vi "UHR-Fleezers Control (host) - 11.8.vi"() -> ()   [LabVIEW 2014] (continued)
        n2364 = call "reset FPGA DMA.vi"("error in"=w4799, "FPGA VI Reference In"=w4800) -> ("error out"=w4795:errorcluster, "FPGA VI Reference Out"=w4796:T19)
        n2365 = xnode "Read/Write Control"("FPGA VI Reference In"=w4796, "error in"=w4795, "AI to FIFO"=w4797, "APD to FIFO"=w4797) -> ("FPGA VI Reference Out"=w4794:T19, "error out"=w4793:errorcluster)
      }
    }
    n2366 = case shown="True" w3436 {
      frame False {
      }
      frame True {
        n2367 = local read "Flush rate (uL/m) P1"() -> (w3827:dbl)
        n2368 = local read "HP1 Flush Time (s)"() -> (w3833:dbl)
        n2369 = local read "DMA Update Period (s)"() -> (w3820:dbl)
        n2370 = Divide(x=w3827, y=60.0) -> (x/y=w3819:dbl)
        n2371 = feedback #4(0.0) -> (w3822:dbl)
        n2372 = Divide(x=w3833, y=w3820) -> (x/y=w3825:dbl)
        n2373 = feedback #5(0) -> (w3831:i32)
        n2374 = Increment(x=w3831) -> (x+1=w3824:i32)
        n2375 = Multiply(x=w3820, y=w3819) -> (x*y=w3818:dbl)
        n2376 = Greater?(x=w3824, y=w3825) -> (0:w3830:bool)
        n2377 = Compound Arithmetic op=MULTIPLY(w3820, w3824, w3819) -> (→"P1 Flush Volume (uL)":dbl)
        n2378 = Divide(x=w3824, y=w3825) -> (x/y=→"P1 Flushing Bar":dbl)
        n2379 = Add(x=w3818, y=w3822) -> (x+y=w3821:dbl)
        "Total Volume\nFlowed P1 (uL)" <- w3821
        n2380 = feedback-in #4(w3821) -> ()
        n2381 = case shown="True" w3830 {
          tunnel: w3824 -> [w3834 _]
          tunnel: [w3834 0] -> w3829
          frame False {
          }
          frame True {
            w3835 = FALSE ("Flushing P1")
            n2382 = local write "Inject Pump 1"(w3835) -> ()
            n2383 = local write "Flushing P1"(w3835) -> ()
            n2384 = property on="Clear Volume P1" class="Bool (strict)"("Val(Sgnl)"=TRUE ("Value (Signaling)")) -> ()  [unwired: 2 in, 2 out]
          }
        }
        n2385 = feedback-in #5(w3829) -> ()
      }
    }
    n2386 = Or(x="Start AOD Scan", y="Trap Raster Scan") -> (x .or. y?=w3671:bool)
    n2387 = case "Start AOM raster scan" shown="True" w3671 {
      tunnel: w3429 -> [w4642 w4652]
      tunnel: w3720 -> [w4641 w4651]
      tunnel: [w4642 w4645] -> w3719
      tunnel: [w4641 w4644] -> w3718
      frame False {
      }
      frame True {
        n2388 = case shown="True" "Restart DMA? (AOD)" {
          tunnel: [w4690 w4692] -> w4646
          tunnel: [w4689 w4691] -> w4647
          tunnel: w4652 -> [w4690 w4694]
          tunnel: w4651 -> [w4689 w4693]
          frame False {
          }
          frame True {
            n2389 = local write "Overflow (data lost)"(FALSE ("Overflow (data lost)")) -> ()
            n2390 = call "reset FPGA DMA.vi"("error in"=w4693, "FPGA VI Reference In"=w4694) -> ("error out"=w4691:errorcluster, "FPGA VI Reference Out"=w4692:T19)
          }
        }
        n2391 = local write "Trap Raster Scan"(FALSE ("Trap Raster Scan")) -> ()
        n2392 = case shown="False" "Move MCL Also?" {
          tunnel: w4647 -> [w4656 w4684]
          tunnel: w4646 -> [w4657 w4685]
          tunnel: [w4655 w4688] -> w4645
          tunnel: [w4654 w4687] -> w4644
          frame False {
            w4653 = TRUE ("AI to FIFO")
            n2393 = xnode "Read/Write Control"("FPGA VI Reference In"=w4657, "error in"=w4656, "AI to FIFO"=w4653, "APD to FIFO"=w4653, "Start scan"=w4653) -> ("FPGA VI Reference Out"=w4655:T19, "error out"=w4654:errorcluster)
          }
          frame True {
            w4681 = FALSE ("1D or 2D Scan?")
            w4686 = TRUE ("AI to FIFO")
            # "Count for MCL loop"
            # "N total cycles"
            # "N steps"
            # "V_int"
            n2394 = local read "Scan Range (nm)"() -> (w4663:dbl)
            n2395 = local read "Number of F/B Scans (AOD)"() -> (w4680:u16)
            n2396 = Sign(1:w4663) -> (0:w4662:dbl)
            n2397 = Compound Arithmetic op=MULTIPLY(w4663, "MCL Step Position Ratio", "MCL/AOM Scale Tweak") -> (w4667:dbl)
            n2398 = Negate(x=w4662) -> (-x=w4659:dbl)
            n2399 = Multiply(x=w4659, y="MCL Step Increment (V_int)") -> (x*y=w4661:dbl)
            n2400 = Divide(x=w4667, y="MCL X Cal (nm/V)") -> (x/y=w4673:dbl)
            n2401 = Multiply(x=32767.0 ("y"), y=w4673) -> (x*y=w4679:dbl)
            n2402 = local read "Total Counts (ticks)"() -> (w4664:u32)
            n2403 = local read "Cycles/step (AOD)"() -> (w4675:u64)
            n2404 = local read "Scan steps (AOD)"() -> (w4676:u64)
            n2405 = Divide(x=w4679, y=10.0) -> (x/y=w4672:dbl)
            n2406 = Divide(x=w4672, y="MCL Step Increment (V_int)") -> (x/y=w4670:dbl)
            n2407 = Absolute Value(x=w4670) -> (abs(x)=w4658:dbl)
            n2408 = Compound Arithmetic op=MULTIPLY(w4676, w4675, w4664) -> (w4671:u64)
            n2409 = local write "wait to reset values"(w4686) -> ()
            n2410 = local write "MCL Scanning"(w4686) -> ()
            n2411 = Divide(x=w4671, y=w4658) -> (x/y=w4668:dbl)
            "MCL Count" <- w4668
            n2412 = xnode "Read/Write Control"("FPGA VI Reference In"=w4685, "error in"=w4684, "Scan steps (MCL)"=w4658, "Number of scans (MCL)"=w4680, "Cycles per step (MCL)"=u64 1, "Scan freq.  increment (MCL)"=w4661, "1D or 2D Scan?"=w4681, "MCL Scan Axis"=w4681, "Cont. Scan (MCL)"=w4681, "MCL count"=w4668) -> ("FPGA VI Reference Out"=w4683:T19, "error out"=w4682:errorcluster)
            n2413 = xnode "Read/Write Control"("FPGA VI Reference In"=w4683, "error in"=w4682, "AI to FIFO"=w4686, "APD to FIFO"=w4686, "Start scan"=w4686, "Start scan (MCL)"=w4686) -> ("FPGA VI Reference Out"=w4688:T19, "error out"=w4687:errorcluster)
          }
        }
        "Raster Scanning..." <- TRUE ("Scanning...")
      }
    }
    n2414 = local read "Flushing P3"() -> (w3437:bool)
    n2415 = case "Keep track of when Harvard Pump 3 is done flushing" shown="True" w3437 {
      frame False {
      }
      frame True {
        n2416 = local read "Flush rate (uL/m) P3"() -> (w3846:dbl)
        n2417 = local read "DMA Update Period (s)"() -> (w3840:dbl)
        n2418 = local read "HP3 Flush Time (s)"() -> (w3854:dbl)
        n2419 = Divide(x=w3846, y=60.0) -> (x/y=w3841:dbl)
        n2420 = feedback #6(0) -> (w3852:i32)
        n2421 = Increment(x=w3852) -> (x+1=w3847:i32)
        n2422 = Divide(x=w3854, y=w3840) -> (x/y=w3848:dbl)
        n2423 = Multiply(x=w3840, y=w3841) -> (x*y=w3839:dbl)
        n2424 = Greater?(x=w3847, y=w3848) -> (0:w3851:bool)
        n2425 = feedback #7(0.0) -> (w3842:dbl)
        n2426 = Compound Arithmetic op=MULTIPLY(w3840, w3847, w3841) -> (→"P3 Flush Volume (uL)":dbl)
        n2427 = case shown="True" w3851 {
          tunnel: w3847 -> [w3855 _]
          tunnel: [w3855 0] -> w3850
          frame False {
          }
          frame True {
            w3856 = FALSE ("Flushing P3")
            n2428 = local write "Inject Pump 3"(w3856) -> ()
            n2429 = local write "Flushing P3"(w3856) -> ()
            n2430 = property on="Clear Volume P3" class="Bool (strict)"("Val(Sgnl)"=TRUE ("Value (Signaling)")) -> ()  [unwired: 2 in, 2 out]
          }
        }
        n2431 = feedback-in #6(w3850) -> ()
        n2432 = Divide(x=w3847, y=w3848) -> (x/y=→"P3 Flushing Bar":dbl)
        n2433 = Add(x=w3839, y=w3842) -> (x+y=w3843:dbl)
        "Total Volume\nFlowed P3 (uL)" <- w3843
        n2434 = feedback-in #7(w3843) -> ()
      }
    }
    n2435 = And(x="Save scans", y=w3671) -> (x .and. y?=w3717:bool)
    n2436 = local read "Flushing samp"() -> (w3430:bool)
    n2437 = case shown="True" w3430 {
      frame False {
      }
      frame True {
        n2438 = local read "DMA Update Period (s)"() -> (w3799:dbl)
        n2439 = local read "Flush rate (mL/m)"() -> (w3811:dbl)
        n2440 = local read "Samp Flush Time (s)"() -> (w3812:dbl)
        n2441 = Divide(x=w3811, y=60.0) -> (x/y=w3798:dbl)
        n2442 = feedback #8(0) -> (w3804:i32)
        n2443 = Increment(x=w3804) -> (x+1=w3803:i32)
        n2444 = Divide(x=w3812, y=w3799) -> (x/y=w3808:dbl)
        n2445 = Multiply(x=w3799, y=w3798) -> (x*y=w3797:dbl)
        n2446 = Greater?(x=w3803, y=w3808) -> (0:w3807:bool)
        n2447 = feedback #9(0.0) -> (w3800:dbl)
        n2448 = Compound Arithmetic op=MULTIPLY(w3799, w3803, w3798) -> (→"Samp Volume (uL)":dbl)
        n2449 = Divide(x=w3803, y=w3808) -> (x/y=→"Samp flush bar":dbl)
        n2450 = case shown="True" w3807 {
          tunnel: [w3813 0] -> w3806
          tunnel: w3803 -> [w3813 _]
          frame False {
          }
          frame True {
            w3816 = FALSE ("Flushing samp")
            n2451 = local write "Sample Channel\nFlow"(w3816) -> ()
            n2452 = local write "Flushing samp"(w3816) -> ()
            n2453 = property on="Clear Volume" class="Bool (strict)"("Val(Sgnl)"=TRUE) -> ()  [unwired: 2 in, 2 out]
          }
        }
        n2454 = feedback-in #8(w3806) -> ()
        n2455 = Add(x=w3797, y=w3800) -> (x+y=w3801:dbl)
        "Total Volume\nFlowed Samp (uL)" <- w3801
        n2456 = feedback-in #9(w3801) -> ()
      }
    }
    n2457 = Compound Arithmetic op=OR("Start MCL Scan", "Confocal\nImage", "Confocal\nLinescan") -> (w3669:bool)
    n2458 = And(x="Save Data (MCL)", y=w3669) -> (x .and. y?=w3716:bool)
    n2459 = case "Start MCL raster scan" shown="True" w3669 {
      tunnel: w3719 -> [w4259 w4275]
      tunnel: w3718 -> [w4258 w4274]
      tunnel: [w4259 w4270] -> w3428
      tunnel: [w4258 w4269] -> w3426
      tunnel: [FALSE w4268] -> w3702
      tunnel: "Start MCL Scan" -> [_ w4263]
      tunnel: "Confocal\nImage" -> [_ w4262]
      tunnel: "Confocal\nLinescan" -> [_ _]
      frame False {
      }
      frame True {
        w4268 = TRUE
        n2460 = case shown="True" "Restart DMA? (MCL)" {
          tunnel: [w4320 w4322] -> w4273
          tunnel: [w4319 w4321] -> w4272
          tunnel: w4275 -> [w4320 w4325]
          tunnel: w4274 -> [w4319 w4324]
          frame False {
          }
          frame True {
            n2461 = call "reset FPGA DMA.vi"("error in"=w4324, "FPGA VI Reference In"=w4325) -> ("error out"=w4321:errorcluster, "FPGA VI Reference Out"=w4322:T19)
            n2462 = local write "Overflow (data lost)"(FALSE ("Overflow (data lost)")) -> ()
          }
        }
        n2463 = case shown="False" w4263 {
          selector: w4263 -> [_ w4279]
          tunnel: w4262 -> [w4278 _]
          tunnel: [w4278 w4279] -> w4261
          frame False {
            n2464 = property on="2D or 1D Scan" class="Bool (strict)"("Val(Sgnl)"=w4278) -> ()  [unwired: 2 in, 2 out]
            n2465 = property on="Confocal\nImage" class="Bool (strict)"("Value"=FALSE ("Start Confocal Map")) -> ()  [unwired: 2 in, 2 out]
          }
          frame True {
          }
        }
        n2466 = local write "MCL Scanning"(w4268) -> ()
        n2467 = local read "AO1"() -> (w4265:dbl)
        n2468 = local read "AO2"() -> (w4264:dbl)
        n2469 = case shown="True" "Center Scan" {
          tunnel: w4273 -> [w4286 w4318]
          tunnel: w4272 -> [w4285 w4317]
          tunnel: [w4284 w4316] -> w4270
          tunnel: [w4283 w4315] -> w4269
          tunnel: [w4281 w4302] -> w4267
          tunnel: [w4280 w4301] -> w4266
          tunnel: w4265 -> [w4281 w4307]
          tunnel: w4264 -> [w4280 w4310]
          tunnel: w4261 -> [_ _]
          frame False {
            w4282 = TRUE ("AI to FIFO")
            n2470 = xnode "Read/Write Control"("FPGA VI Reference In"=w4286, "error in"=w4285, "AI to FIFO"=w4282, "APD to FIFO"=w4282, "Start scan (MCL)"=w4282) -> ("FPGA VI Reference Out"=w4284:T19, "error out"=w4283:errorcluster)
          }
          frame True {
            w4314 = TRUE ("AI to FIFO")
            n2471 = local read "Scan steps (MCL)"() -> (w4293:u64)
            n2472 = local read "Scan lines (y)"() -> (w4289:u64)
            n2473 = local read "Fast Scan Dir"() -> (w4300:bool)
            n2474 = local read "Actual MCL Inc (V)"() -> (w4290:dbl)
            n2475 = Decrement(x=w4289) -> (x-1=w4288:u64)
            n2476 = Decrement(x=w4293) -> (x-1=w4292:u64)
            n2477 = Multiply(x=w4290, y=w4288) -> (x*y=w4287:dbl)
            n2478 = Divide(x=w4287, y=2.0) -> (x/y=w4297:dbl)
            n2479 = Multiply(x=w4290, y=w4292) -> (x*y=w4291:dbl)
            n2480 = Divide(x=w4291, y=2.0) -> (x/y=w4296:dbl)
            n2481 = Select(t=w4296, s=w4300, f=w4297) -> (s? t:f=w4295:dbl)
            n2482 = Select(t=w4297, s=w4300, f=w4296) -> (s? t:f=w4299:dbl)
            n2483 = Subtract(x=w4307, y=w4299) -> (x-y=w4298:dbl)
            n2484 = Subtract(x=w4310, y=w4295) -> (x-y=w4294:dbl)
            n2485 = local read "2D or 1D Scan"() -> (w4312:bool)
            n2486 = Not(x=w4300) -> (.not. x?=w4306:bool)
            n2487 = Not(x=w4312) -> (.not. x?=w4308:bool)
            n2488 = And(x=w4300, y=w4308) -> (x .and. y?=w4309:bool)
            n2489 = And(x=w4308, y=w4306) -> (x .and. y?=w4311:bool)
            n2490 = Select(t=w4310, s=w4311, f=w4294) -> (s? t:f=w4301:dbl)
            n2491 = Select(t=w4307, s=w4309, f=w4298) -> (s? t:f=w4302:dbl)
            n2492 = call "Volt to I16.vi"("Voltage In"=w4302) -> ("I16 Voltage Out"=w4305:i16)
            n2493 = call "Volt to I16.vi"("Voltage In"=w4301) -> ("I16 Voltage Out"=w4304:i16)
            n2494 = xnode "Read/Write Control"("FPGA VI Reference In"=w4318, "error in"=w4317, "AI to FIFO"=w4314, "APD to FIFO"=w4314, "Start scan (MCL)"=w4314, "AO1"=w4305, "AO2"=w4304) -> ("FPGA VI Reference Out"=w4316:T19, "error out"=w4315:errorcluster)
          }
        }
        "Initial Y" <- w4267
        "Initial X" <- w4266
        n2495 = local write "Tab Control 6"(T3."Imaging" ("Tab Control 6")) -> ()
        "wait to reset values" <- w4268
      }
    }
    n2496 = case shown="True" "Wiggle" {
      selector: "Wiggle" -> [w3770 _]
      tunnel: w3428 -> [w3772 w3785]
      tunnel: [w3769 w3788] -> w3427
      tunnel: w3426 -> [w3771 w3783]
      tunnel: [w3768 w3787] -> w3425
      frame False {
        n2497 = xnode "Read/Write Control"("FPGA VI Reference In"=w3772, "error in"=w3771, "Wiggle trap 1"=w3770) -> ("FPGA VI Reference Out"=w3769:T19, "error out"=w3768:errorcluster)
      }
      frame True {
        w3777 = FALSE ("Abort wiggle")
        w3781 = TRUE
        n2498 = local read "Restart DMA? (AOD)"() -> (w3786:bool)
        n2499 = case shown="True" w3786 {
          tunnel: w3785 -> [w3790 w3795]
          tunnel: [w3790 w3794] -> w3784
          tunnel: w3783 -> [w3789 w3793]
          tunnel: [w3789 w3792] -> w3782
          frame False {
          }
          frame True {
            n2500 = local write "Overflow (data lost)"(FALSE) -> ()
            n2501 = call "reset FPGA DMA.vi"("error in"=w3793, "FPGA VI Reference In"=w3795) -> ("error out"=w3792:errorcluster, "FPGA VI Reference Out"=w3794:T19)
          }
        }
        n2502 = local write "Wiggle"(FALSE) -> ()
        n2503 = xnode "Read/Write Control"("FPGA VI Reference In"=w3784, "error in"=w3782, "AI to FIFO"=w3781, "APD to FIFO"=w3781, "Wiggle trap 1"="Wiggle T1", "Wiggle freq 1 (Hz)"="Wiggle freq 1 (Hz)", "Wiggle amp 1"="Wiggle amp 1 (units?)", "Abort wiggle 1"=w3777, "Wiggle trap 2"="Wiggle T2", "Abort wiggle 2"=w3777, "Wiggle freq 2 (Hz)"="Wig Freq 2 (Hz)", "Wiggle amp 2"="Wig amp 2") -> ("FPGA VI Reference Out"=w3788:T19, "error out"=w3787:errorcluster)
      }
    }
    n2504 = local read "Trap Pos Elements/DMA read"() -> (w3559:u32)
    n2505 = local read "Trap AI Elements/DMA read"() -> (w3632:u32)
    n2506 = local read "APD Elements/DMA read"() -> (w3598:u32)
    n2507 = xnode "Get APD Data"("FPGA VI Reference In"=w3427, "error in"=w3425, "Number of Elements"=w3598, "Timeout (ms)"=-1) -> ("Data"=w3597:u32[], "Elements Remaining"=→"APD FIFO Elements Remaining":u32)  [unwired: 2 out]
    n2508 = xnode "Invoke Method"("FPGA VI Reference In"=w3427, "error in"=w3425, "Number of Elements"=w3559, "Timeout (ms)"=-1) -> ("Data"=w3523:u16[], "Elements Remaining"=→"Trap Pos FIFO El Remaining":u32)  [unwired: 2 out]
    n2509 = xnode "Get Trap Data"("FPGA VI Reference In"=w3427, "error in"=w3425, "Number of Elements"=w3632, "Timeout (ms)"=-1 ("Timeout")) -> ("FPGA VI Reference Out"=w3458:T19, "error out"=w3457:errorcluster, "Data"=w3524:i16[], "Elements Remaining"=w3762:u32)
    "FIFO El. Rem." <- w3762
    n2510 = local read "Trap AI FIFO Depth"() -> (w3764:u32)
    n2511 = Subtract(x=w3764, y=w3632) -> (x-y=w3763:u32)
    n2512 = Decimate 1D Array(w3523) -> (w3520:u16[], w3522:u16[], w3521:u16[])
    n2513 = Divide(x=w3762, y=w3763) -> (x/y=w3761:dbl)
    "Buffer Status" <- w3761
    n2514 = To Unsigned Long Integer(number=w3520) -> (unsigned 32bit integer=w3519:u32[])
    n2515 = Join Numbers(hi=w3522, lo=w3521) -> ((hi.lo)=w3518:u32[])
    n2516 = Equal?(x=w3761, y=1.0) -> (x = y?=w3759:bool)
    n2517 = Join Numbers(hi=w3519, lo=w3518) -> ((hi.lo)=w3512:u64[])
    n2518 = call "IR AOM word to freq - vec.vi"("Frequency Word In (double vec)"=w3512) -> ("Frequency Out"=w3558:dbl[])
    n2519 = case "Alert buffer overflow" shown="True" w3759 {
      frame False {
      }
      frame True {
        n2520 = call <vilib>:"Beep.vi"() -> ()  [unwired: 3 in, 9 out]
        "Overflow (data lost)" <- TRUE ("Overflow (data lost)")
      }
    }
    n2521 = Decimate 1D Array(w3558) -> (w3557:dbl[], w3556:dbl[])
    n2522 = Build Array(w3557, w3556) -> (w3555:dbl[][])
    n2523 = local read "Trap Sets"() -> (w3631:u32)
    n2524 = case "Deinterlace trap data, average down PSD" shown="2" w3631 {
      tunnel: w3524 -> [w4355 w4420]
      tunnel: [w4352 w4417] -> w3624
      tunnel: [w4355 w4419] -> w3515
      tunnel: "Detector Type" -> [w4354 w4415]
      tunnel: [w4353 w4418] -> w3623
      tunnel: [w4351 w4416] -> w3736
      frame 1, Default {
        n2525 = Divide(x=w4355, y=3276.7) -> (x/y=w4356:dbl[])
        n2526 = Decimate 1D Array(w4356) -> (w4365:dbl[], w4364:dbl[], w4363:dbl[], w4362:dbl[], w4361:dbl[], w4360:dbl[], w4359:dbl[], w4358:dbl[])
        n2527 = case shown="\"IR-QPD + PSD + FB-QPD position\"" w4354 {
          tunnel: w4365 -> [w4389 w4414]
          tunnel: w4364 -> [w4388 w4413]
          tunnel: w4363 -> [w4373 w4391]
          tunnel: w4362 -> [w4374 w4401]
          tunnel: w4361 -> [w4387 w4412]
          tunnel: w4360 -> [w4386 w4411]
          tunnel: w4359 -> [w4370 w4392]
          tunnel: w4358 -> [w4369 w4390]
          tunnel: [w4368 w4398] -> w4353
          tunnel: [w4367 w4397] -> w4352
          tunnel: [w4366 w4396] -> w4351
          frame "IR-QPD + PSD + FB-QPD", Default {
            w4366 = 0  # Channel pattern
            n2528 = Divide(x=w4389, y=w4374) -> (x/y=w4376:dbl[])
            n2529 = Divide(x=w4388, y=w4374) -> (x/y=w4375:dbl[])
            n2530 = Divide(x=w4387, y=w4370) -> (x/y=w4372:dbl[])
            n2531 = Divide(x=w4386, y=w4369) -> (x/y=w4371:dbl[])
            n2532 = Build Array(w4376, w4375, w4374, w4373, w4372, w4371, w4370, w4369) -> (w4367:dbl[][])
            n2533 = Bundle("T1 Y", "T1 X", "T1 Sum", "FB Sum", "PSD Y", "PSD X", "PSD Y Sum", "PSD X Sum") -> (w4385:T41)  [unwired: 1 out]
            n2534 = Cluster To Array(cluster=w4385) -> (array=w4368:string[])
          }
          frame "IR-QPD + PSD + FB-QPD position" {
            w4396 = 3  # Channel pattern
            n2535 = Negate(x=w4392) -> (-x=w4393:dbl[])
            n2536 = Divide(x=w4414, y=w4401) -> (x/y=w4403:dbl[])
            n2537 = Divide(x=w4413, y=w4401) -> (x/y=w4402:dbl[])
            n2538 = Divide(x=w4412, y=w4392) -> (x/y=w4400:dbl[])
            n2539 = Divide(x=w4411, y=w4393) -> (x/y=w4399:dbl[])
            n2540 = Build Array(w4403, w4402, w4401, w4390, w4391, w4400, w4399, w4392) -> (w4397:dbl[][])
            n2541 = Bundle("T1 Y", "T1 X", "T1 Sum", "FB X", "FB Sum", "PSD Y", "PSD X", "PSD Y Sum") -> (w4410:T41)  [unwired: 1 out]
            n2542 = Cluster To Array(cluster=w4410) -> (array=w4398:string[])
          }
        }
      }
      frame 2 {
        n2543 = case shown="\"IR-QPD + PSD + FB-QPD\", Default" w4415 {
          tunnel: w4420 -> [w4482 w4549 w4620]
          tunnel: [w4421 w4540 w4551] -> w4419
          tunnel: [w4448 w4531 w4598] -> w4418
          tunnel: [w4447 w4494 w4565] -> w4417
          tunnel: [w4441 w4529 w4596] -> w4416
          frame "IR-QPD + PSD + FB-QPD", Default {
            w4441 = 1  # Channel pattern
            # "time average x2 the 4th signal and the 4 psd signals (detection laser)"
            # "deinterlace 3 signals from qpd"
            n2544 = Decimate 1D Array(w4482) -> (w4481:i16[], w4480:i16[], w4446:i16[], w4479:i16[], w4469:i16[], w4467:i16[], w4466:i16[], w4464:i16[])
            n2545 = Decimate 1D Array(w4446) -> (w4445:i16[], w4444:i16[])
            n2546 = Decimate 1D Array(w4481) -> (w4478:i16[], w4450:i16[])
            n2547 = Decimate 1D Array(w4480) -> (w4477:i16[], w4475:i16[])
            n2548 = Decimate 1D Array(w4479) -> (w4476:i16[], w4474:i16[])
            n2549 = call "downsample 1D array - double.vi"("Ave N"=2.0, "Array In"=w4469) -> ("Array Out"=w4468:dbl[])  [unwired: 1 out]
            n2550 = call "downsample 1D array - double.vi"("Ave N"=2.0, "Array In"=w4467) -> ("Array Out"=w4449:dbl[])  [unwired: 1 out]
            n2551 = call "downsample 1D array - double.vi"("Ave N"=2.0, "Array In"=w4466) -> ("Array Out"=w4465:dbl[])  [unwired: 1 out]
            n2552 = call "downsample 1D array - double.vi"("Ave N"=2.0, "Array In"=w4464) -> ("Array Out"=w4463:dbl[])  [unwired: 1 out]
            n2553 = Interleave 1D Arrays(w4478, w4477, w4476, w4450, w4475, w4474, w4445, w4444, w4468, w4449, w4465, w4463) -> (w4462:dbl[])
            n2554 = Divide(x=w4462, y=3276.7) -> (x/y=w4461:dbl[])
            n2555 = Decimate 1D Array(w4461) -> (w4460:dbl[], w4459:dbl[], w4458:dbl[], w4457:dbl[], w4456:dbl[], w4455:dbl[], w4443:dbl[], w4442:dbl[], w4454:dbl[], w4453:dbl[], w4452:dbl[], w4451:dbl[])
            n2556 = Divide(x=w4460, y=w4458) -> (x/y=w4428:dbl[])
            n2557 = Divide(x=w4459, y=w4458) -> (x/y=w4427:dbl[])
            n2558 = Divide(x=w4457, y=w4455) -> (x/y=w4426:dbl[])
            n2559 = Divide(x=w4456, y=w4455) -> (x/y=w4425:dbl[])
            n2560 = Divide(x=w4454, y=w4452) -> (x/y=w4424:dbl[])
            n2561 = Divide(x=w4453, y=w4451) -> (x/y=w4423:dbl[])
            n2562 = Build Array(w4428, w4427, w4458, w4426, w4425, w4455, w4443, w4442, w4424, w4423, w4452, w4451) -> (w4447:dbl[][])
            n2563 = Bundle("T1 Y", "T1 X", "T1 Sum", "T2 Y", "T2 X", "T2 Sum", "T1 FB Sum", "T2 FB Sum", "PSD Y", "PSD X", "PSD Y Sum", "PSD X Sum") -> (w4429:T42)  [unwired: 1 out]
            n2564 = To Word Integer(number=w4462) -> (16bit integer=w4421:i16[])
            n2565 = Cluster To Array(cluster=w4429) -> (array=w4448:string[])
          }
          frame "IR-QPD + PSD + FB-QPD X position" {
            w4529 = 2  # Channel pattern
            # "time average x2 the 3 psd signals (detection laser)"
            # "deinterlace 3 signals from qpds"
            n2566 = Decimate 1D Array(w4549) -> (w4548:i16[], w4547:i16[], w4530:i16[], w4546:i16[], w4492:i16[], w4489:i16[], w4486:i16[], w4517:i16[])
            n2567 = Decimate 1D Array(w4530) -> (w4515:i16[], w4513:i16[])
            n2568 = Decimate 1D Array(w4548) -> (w4545:i16[], w4532:i16[])
            n2569 = Decimate 1D Array(w4547) -> (w4544:i16[], w4542:i16[])
            n2570 = Decimate 1D Array(w4546) -> (w4543:i16[], w4541:i16[])
            n2571 = Decimate 1D Array(w4517) -> (w4516:i16[], w4514:i16[])
            n2572 = call "downsample 1D array - I16.vi"("Ave N"=2.0, "Array In"=w4492) -> ("Array Out"=w4490:i16[])  [unwired: 1 in]
            n2573 = call "downsample 1D array - I16.vi"("Ave N"=2.0, "Array In"=w4486) -> ("Array Out"=w4484:i16[])  [unwired: 1 in]
            n2574 = call "downsample 1D array - I16.vi"("Ave N"=2.0, "Array In"=w4489) -> ("Array Out"=w4487:i16[])  [unwired: 1 in]
            n2575 = Interleave 1D Arrays(w4545, w4544, w4543, w4532, w4542, w4541, w4516, w4515, w4514, w4513, w4490, w4487, w4484) -> (w4540:i16[])
            n2576 = Divide(x=w4540, y=3276.7) -> (x/y=w4539:dbl[])
            n2577 = Decimate 1D Array(w4539) -> (w4538:dbl[], w4537:dbl[], w4536:dbl[], w4535:dbl[], w4534:dbl[], w4533:dbl[], w4505:dbl[], w4503:dbl[], w4502:dbl[], w4500:dbl[], w4499:dbl[], w4498:dbl[], w4495:dbl[])
            n2578 = Negate(x=w4495) -> (-x=w4493:dbl[])
            n2579 = Divide(x=w4499, y=w4495) -> (x/y=w4497:dbl[])
            n2580 = Divide(x=w4498, y=w4493) -> (x/y=w4496:dbl[])
            n2581 = Divide(x=w4538, y=w4536) -> (x/y=w4521:dbl[])
            n2582 = Divide(x=w4537, y=w4536) -> (x/y=w4520:dbl[])
            n2583 = Divide(x=w4535, y=w4533) -> (x/y=w4519:dbl[])
            n2584 = Divide(x=w4534, y=w4533) -> (x/y=w4518:dbl[])
            n2585 = Divide(x=w4505, y=w4503) -> (x/y=w4504:dbl[])
            n2586 = Divide(x=w4502, y=w4500) -> (x/y=w4501:dbl[])
            n2587 = Build Array(w4521, w4520, w4536, w4519, w4518, w4533, w4504, w4503, w4501, w4500, w4497, w4496, w4495) -> (w4494:dbl[][])
            n2588 = Bundle("T1 Y", "T1 X", "T1 Sum", "T2 Y", "T2 X", "T2 Sum", "T1 FB X", "T1 FB Sum", "T2 FB X", "T2 FB Sum", "PSD Y", "PSD X", "PSD Y Sum") -> (w4522:T43)  [unwired: 1 out]
            n2589 = Cluster To Array(cluster=w4522) -> (array=w4531:string[])
          }
          frame "IR-QPD + PSD + FB-QPD XY positions" {
            w4596 = 4  # Channel pattern
            # "time average x2 the 3 psd signals (detection laser)"
            # "deinterlace 3 signals from qpds"
            n2590 = Decimate 1D Array(w4620) -> (w4619:i16[], w4618:i16[], w4597:i16[], w4617:i16[], w4563:i16[], w4609:i16[], w4608:i16[], w4585:i16[])
            n2591 = Decimate 1D Array "Feedback Sum"(w4597) -> (w4581:i16[], w4579:i16[])
            n2592 = Decimate 1D Array "QPD Y"(w4619) -> (w4616:i16[], w4599:i16[])
            n2593 = Decimate 1D Array "QPD X"(w4618) -> (w4615:i16[], w4613:i16[])
            n2594 = Decimate 1D Array "Feedback Y"(w4563) -> (w4562:i16[], w4561:i16[])
            n2595 = Decimate 1D Array "QPD Sum"(w4617) -> (w4614:i16[], w4612:i16[])
            n2596 = Decimate 1D Array "Feedback X"(w4585) -> (w4582:i16[], w4580:i16[])
            n2597 = call "downsample 1D array - double.vi"("Ave N"=2.0, "Array In"=w4609) -> ("Array Out"=w4584:dbl[])  [unwired: 1 out]
            n2598 = call "downsample 1D array - double.vi"("Ave N"=2.0, "Array In"=w4608) -> ("Array Out"=w4583:dbl[])  [unwired: 1 out]
            n2599 = Interleave 1D Arrays(w4616, w4615, w4614, w4599, w4613, w4612, w4562, w4582, w4581, w4561, w4580, w4579, w4584, w4583) -> (w4607:dbl[])
            n2600 = Divide(x=w4607, y=3276.7) -> (x/y=w4606:dbl[])
            n2601 = Decimate 1D Array(w4606) -> (w4605:dbl[], w4604:dbl[], w4603:dbl[], w4602:dbl[], w4601:dbl[], w4600:dbl[], w4558:dbl[], w4572:dbl[], w4556:dbl[], w4557:dbl[], w4570:dbl[], w4554:dbl[], w4568:dbl[], w4566:dbl[])
            n2602 = Negate(x=w4566) -> (-x=w4564:dbl[])
            n2603 = Divide(x=w4568, y=w4564) -> (x/y=w4567:dbl[])
            n2604 = Divide(x=w4557, y=w4554) -> (x/y=w4553:dbl[])
            n2605 = Divide(x=w4558, y=w4556) -> (x/y=w4555:dbl[])
            n2606 = Divide(x=w4605, y=w4603) -> (x/y=w4589:dbl[])
            n2607 = Divide(x=w4604, y=w4603) -> (x/y=w4588:dbl[])
            n2608 = Divide(x=w4602, y=w4600) -> (x/y=w4587:dbl[])
            n2609 = Divide(x=w4601, y=w4600) -> (x/y=w4586:dbl[])
            n2610 = Divide(x=w4572, y=w4556) -> (x/y=w4571:dbl[])
            n2611 = Divide(x=w4570, y=w4554) -> (x/y=w4569:dbl[])
            n2612 = Build Array(w4589, w4588, w4603, w4587, w4586, w4600, w4555, w4571, w4556, w4553, w4569, w4554, w4567, w4566) -> (w4565:dbl[][])
            n2613 = Bundle("T1 Y", "T1 X", "T1 Sum", "T2 Y", "T2 X", "T2 Sum", "T1 FB Y", "T1 FB X", "T1 FB Sum", "T2 FB Y", "T2 FB X", "T2 FB Sum", "PSD X", "PSD Y Sum") -> (w4552:T44)  [unwired: 1 out]
            n2614 = To Word Integer(number=w4607) -> (16bit integer=w4551:i16[])
            n2615 = Cluster To Array(cluster=w4552) -> (array=w4598:string[])
          }
        }
      }
    }
    "AI labels" <- w3623
    n2616 = Decimate 1D Array(w3597) -> (w3621:u32[], w3565:u32[])
    n2617 = local read "DMA Update Period (s)"() -> (w3633:dbl)
    n2618 = Build Array(w3621, w3565) -> (w3699:u32[][])
    n2619 = local read "Data Period (s)"() -> (w3474:dbl)
    n2620 = local read "BD 1 Frequency 2 (MHz)"() -> (w3507:dbl)
    n2621 = local read "BD 1 Frequency 1 (MHz)"() -> (w3508:dbl)
    n2622 = Decimate 1D Array(w3515) -> (w3538:i16[], w3537:i16[], w3535:i16[], w3534:i16[])  [unwired: 9 out]
    n2623 = To Double Precision Float(number=w3699) -> (double precision float=w3700:dbl[][])
    n2624 = local read "APD Integration Time (s)"() -> (w3578:dbl)
    n2625 = Multiply(x=w3474, y="Trap Pos. Disp. Downsample") -> (x*y=w3472:dbl)
    n2626 = Divide(x=w3538, y=w3537) -> (x/y=w3539:dbl[])
    n2627 = Divide(x=w3535, y=w3534) -> (x/y=w3536:dbl[])
    n2628 = feedback #10(0.0) -> (w3552:dbl)
    n2629 = Add(x=w3633, y=w3552) -> (x+y=w3738:dbl)
    n2630 = feedback-in #10(w3738) -> ()
    n2631 = local read "AOM X Cal (nm/MHz)"() -> (w3505:dbl)
    n2632 = To Time Stamp(1:w3552) -> (0:w3551:timestamp)
    n2633 = Split 1D Array(array=w3539, index="N El. to Ave.") -> (second subarray=w3542:dbl[])  [unwired: 1 out]
    n2634 = Split 1D Array(array=w3536, index="N El. to Ave.") -> (second subarray=w3541:dbl[])  [unwired: 1 out]
    n2635 = Multiply(x=w3474, y="Trap Disp. Downsample") -> (x*y=w3553:dbl)
    "Display Period (s)" <- w3553
    n2636 = for "Trap AI" {
      tunnel: [w4350] -> w3732 mode=indexing
      tunnel: w3551 -> [w4340]
      tunnel: "Trap Disp. Downsample" -> [w4348]
      tunnel: w3624 -> [w4346] mode=indexing
      tunnel: w3474 -> [w4345]
      tunnel: w3623 -> [w4344] mode=indexing
      tunnel: w3550 -> [w4343]
      tunnel: [w4342] -> w3589 mode=indexing
      tunnel: w3553 -> [w4341]
      workers-P: _ -> [_]
      n2637 = Bundle By Name("Y"=w4346, "dt"=w4345) -> (w4347:waveform(dbl))  [unwired: 1 out]
      n2638 = Set Waveform Attribute(5:w4344, 6:w4343, 7:w4347) -> (3:w4342:waveform(dbl))  [unwired: 1 in, 2 out]
      n2639 = call "downsample 1D array - double.vi"("Ave N"=w4348, "Array In"=w4346) -> ("Array Out"=w4349:dbl[])  [unwired: 1 out]
      n2640 = Bundle By Name(cluster=w4342, "t0"=w4340, "Y"=w4349, "dt"=w4341) -> (w4350:waveform(dbl))
    }
    n2641 = Bundle("BD 1 Frequency 1 (MHz)"=w3508, "BD 1 Frequency 2 (MHz)"=w3507) -> (w3509:T45)  [unwired: 1 out]
    n2642 = call-poly <vilib>:"Mean.vi"("X"=w3541) -> ("mean"=w3529:dbl)  [unwired: 1 out]
    n2643 = call-poly <vilib>:"Mean.vi"("X"=w3542) -> ("mean"=w3530:dbl)  [unwired: 1 out]
    n2644 = Reciprocal(x=w3553) -> (1/x=→"Trap Disp. Freq. (Hz)":dbl)
    n2645 = Cluster To Array(cluster=w3509) -> (array=w3506:dbl[])
    n2646 = local read "Trap X AI1 (DMA)"() -> (w3540:T13)
    n2647 = local read "Data points/scans (MCL)"() -> (w3711:dbl)
    n2648 = To Fixed-Point(number=w3529) -> (fixed-point=w3527:fxp<+/-,16,1>)  [unwired: 1 in]
    n2649 = To Fixed-Point(number=w3530) -> (fixed-point=w3528:fxp<+/-,16,1>)  [unwired: 1 in]
    n2650 = Bundle("Trap 1 Pos.", "Trap 2 Pos.") -> (w3549:cluster{string, string})  [unwired: 1 out]
    n2651 = Bundle By Name(cluster=w3540, "Set 1"=w3528, "Set 2"=w3527) -> (→"Trap X AI1 (DMA)":T13)
    n2652 = Cluster To Array(cluster=w3549) -> (array=w3546:string[])
    n2653 = Bundle("APD 1", "APD 2") -> (w3731:cluster{string, string})  [unwired: 1 out]
    n2654 = Select(t=-1.0, s="Negate Y Axis", f=1.0) -> (s? t:f=w3491:dbl)
    n2655 = for "Trap Position" {
      tunnel: w3555 -> [w3984] mode=indexing
      tunnel: "Trap Pos. Disp. Downsample" -> [w3983]
      tunnel: w3472 -> [w3981]
      tunnel: w3551 -> [w3980]
      tunnel: w3550 -> [w3978]
      tunnel: w3546 -> [w3977] mode=indexing
      tunnel: [w3976] -> w3461 mode=indexing
      tunnel: w3506 -> [w3974] mode=indexing
      tunnel: w3505 -> [w3972]
      tunnel: w3491 -> [w3971]
      n2656 = call "downsample 1D array - double.vi"("Ave N"=w3983, "Array In"=w3984) -> ("Array Out"=w3982:dbl[])  [unwired: 1 out]
      n2657 = Subtract(x=w3982, y=w3974) -> (x-y=w3975:dbl[])
      n2658 = Multiply(x=w3972, y=w3975) -> (x*y=w3973:dbl[])
      n2659 = Multiply(x=w3971, y=w3973) -> (x*y=w3970:dbl[])
      n2660 = Bundle By Name("Y"=w3970, "dt"=w3981, "t0"=w3980) -> (w3979:waveform(dbl))  [unwired: 1 out]
      n2661 = Set Waveform Attribute(5:w3977, 6:w3978, 7:w3979) -> (3:w3976:waveform(dbl))  [unwired: 1 in, 2 out]
    }
    n2662 = Cluster To Array(cluster=w3731) -> (array=w3728:string[])
    n2663 = for "APD" {
      tunnel: w3700 -> [w4329] mode=indexing
      tunnel: w3578 -> [w4337]
      tunnel: [w4333] -> w3585 mode=indexing
      tunnel: "APD Disp. Scale" -> [w4334]
      tunnel: w3550 -> [w4332]
      tunnel: w3728 -> [w4331] mode=indexing
      tunnel: "APD Disp. Downsample" -> [w4327]
      tunnel: [w4330] -> w3727
      workers-P: _ -> [_]
      tunnel: w3551 -> [w4326]
      n2664 = call "integrate 1D array interval - double.vi"("Ave N"=w4327, "Array In"=w4329) -> ("Array Out"=w4328:dbl[])  [unwired: 1 out]
      n2665 = Multiply(x=w4337, y=w4327) -> (x*y=w4330:dbl)
      n2666 = Divide(x=w4328, y=w4334) -> (x/y=w4335:dbl[])
      n2667 = Bundle By Name("t0"=w4326, "Y"=w4335, "dt"=w4330) -> (w4336:waveform(dbl))  [unwired: 1 out]
      n2668 = Set Waveform Attribute(5:w4331, 6:w4332, 7:w4336) -> (3:w4333:waveform(dbl))  [unwired: 1 in, 2 out]
    }
    "APD Display Period (s)" <- w3727
    n2669 = Reciprocal(x=w3727) -> (1/x=→"APD Display Freq. (Hz)":dbl)
    n2670 = local read "Display Period (s)"() -> (w3609:dbl)
    n2671 = Increment(x=w3711) -> (x+1=w3712:dbl)
    n2672 = To Double Precision Float(number=w3621) -> (double precision float=w3620:dbl[])
    n2673 = Index Array(array=w3461, index=0) -> (element=w3465:waveform(dbl))
    n2674 = Index Array(array=w3461, index=1) -> (element=w3460:waveform(dbl))
    n2675 = feedback #11(w3712) -> (w3715:dbl)
    n2676 = Select(t=0, s=w3702, f=w3715) -> (s? t:f=w3708:dbl)
    n2677 = Array Size(array=w3620) -> (size(s)=w3714:i32)
    n2678 = Add(x=w3714, y=w3708) -> (x+y=w3709:dbl)
    n2679 = Unbundle By Name(w3465) -> ("Y"=w3466:dbl[])
    n2680 = feedback #12(w3621) -> (w3698:u32[])
    n2681 = Build Array (concatenate)(w3698, w3621) -> (w3695:u32[])
    n2682 = feedback #13(w3565) -> (w3584:u32[])
    n2683 = Divide(x="Bead Sep. Int. Time (s)", y=w3609) -> (x/y=w3501:dbl)
    n2684 = Build Array (concatenate)(w3584, w3565) -> (w3583:u32[])
    n2685 = Add(x=w3466, y="FB Trap Pos Offset") -> (x+y=w3464:dbl[])
    "T1 x pos data" <- w3464
    n2686 = Greater?(x=w3709, y=w3711) -> (0:w3710:bool)
    n2687 = feedback #14(w3464) -> (w3503:dbl[])
    n2688 = Build Array (concatenate)(w3464, w3503) -> (w3502:dbl[])
    n2689 = Bundle By Name(cluster=w3465, "Y"=w3464) -> (w3463:waveform(dbl))
    n2690 = Select(t=w3708, s=w3710, f=w3709) -> (s? t:f=w3707:dbl)
    n2691 = feedback-in #11(w3707) -> ()
    n2692 = Array Size(array=w3695) -> (size(s)=w3692:i32)
    n2693 = Array Size(array=w3621) -> (size(s)=w3694:i32)
    n2694 = local read "MCL Scanning"() -> (w3705:bool)
    n2695 = local read "APD Integration Time (s)"() -> (w3592:dbl)
    n2696 = Bundle(w3463, w3460) -> (w3459:cluster{waveform(dbl), waveform(dbl)})  [unwired: 1 out]
    n2697 = Build Array (concatenate)(w3585, w3732) -> (w3587:waveform(dbl)[])
    "All Signals" <- w3587
    n2698 = Split 1D Array(array=w3502, index=w3501) -> (first subarray=w3495:dbl[])  [unwired: 1 out]
    n2699 = feedback-in #14(w3495) -> ()
    n2700 = Multiply(x=w3694, y="APD Ave N") -> (x*y=w3693:dbl)
    n2701 = Greater?(x=w3692, y=w3693) -> (0:w3696:bool)
    n2702 = Not(x=w3710) -> (.not. x?=w3704:bool)
    n2703 = Cluster To Array(cluster=w3459) -> (array=w3435:waveform(dbl)[])
    "Trap Positions" <- w3435
    n2704 = To Double Precision Float(number=w3565) -> (double precision float=w3564:dbl[])
    n2705 = call-poly <vilib>:"Mean.vi"("X"=w3495) -> ("mean"=w3494:dbl)  [unwired: 1 out]
    "Mean T1 Position (nm)" <- w3494
    n2706 = Subtract(x=w3495, y=w3494) -> (x-y=w3500:dbl[])
    n2707 = Square(x=w3500) -> (x^2=w3499:dbl[])
    n2708 = And(x=w3704, y=w3705) -> (x .and. y?=w3706:bool)
    n2709 = call-poly <vilib>:"Mean.vi"("X"=w3499) -> ("mean"=w3498:dbl)  [unwired: 1 out]
    n2710 = case shown="True" w3696 {
      tunnel: w3695 -> [w4109 w4116]
      tunnel: [w4109 w4114] -> w3638
      tunnel: w3693 -> [_ w4111]
      tunnel: w3692 -> [_ w4115]
      tunnel: w3583 -> [w4108 w4113]
      tunnel: [w4108 w4110] -> w3580
      frame False {
      }
      frame True {
        n2711 = Subtract(x=w4115, y=w4111) -> (x-y=w4112:dbl)
        n2712 = Array Subset(array=w4116, index=w4112, length=w4111) -> (w4114:u32[])
        n2713 = Array Subset(array=w4113, index=w4112, length=w4111) -> (w4110:u32[])
      }
    }
    n2714 = feedback-in #12(w3638) -> ()
    n2715 = feedback-in #13(w3580) -> ()
    n2716 = Square Root(x=w3498) -> (sqrt(x)=w3497:dbl)
    n2717 = Or(x=w3706, y=w3702) -> (x .or. y?=w3703:bool)
    n2718 = Equal?(x="Tab Control 6", y=T35."High Res Display") -> (x = y?=w3627:bool)
    n2719 = Multiply(x="APD Disp. Scale", y=w3585) -> (x*y=w3594:waveform(dbl)[])
    n2720 = Multiply(x=10.0, y=w3497) -> (x*y=→"Trap 1 Position RMS (A)":dbl)
    n2721 = Multiply(x="APD Disp. Downsample", y=w3592) -> (x*y=w3590:dbl)
    n2722 = Divide(x=w3594, y=w3590) -> (x/y=w3562:waveform(dbl)[])
    n2723 = case "For displaying the high resolution display (no downsampling)" shown="True" w3627 {
      tunnel: w3589 -> [_ w4009]
      frame False {
      }
      frame True {
        n2724 = Index Array(array=w4009, index="High Res. Display") -> (element=w4010:waveform(dbl))
        n2725 = call <vilib>:"Std Deviation and Variance.vi"("X"=w4010) -> ("mean"=w4017:dbl, "standard deviation"=w4022:dbl)  [unwired: 1 in, 1 out]
        "Mean Intensity" <- w4017
        "Sigma" <- w4022
        n2726 = Subtract(x=w4010, y=w4017) -> (x-y=w4016:waveform(dbl))
        n2727 = Select(t=w4016, s="Subtract mean", f=w4010) -> (s? t:f=→"1 Channel":waveform(dbl))
        n2728 = Divide(x=w4022, y=w4017) -> (x/y=→"Sigma/Mean":dbl)
        n2729 = feedback #15(1) -> (w4011:i32)
        n2730 = Greater Or Equal?(x=w4011, y="Slow mean N ave.") -> (x >= y?=w4024:bool)
        n2731 = Increment(x=w4011) -> (x+1=w4026:i32)
        n2732 = Select(t=1, s=w4024, f=w4026) -> (s? t:f=w4013:i32)
        n2733 = feedback-in #15(w4013) -> ()
        n2734 = feedback #16() -> (w4014:waveform(dbl))  [unwired: 1 out]
        n2735 = case shown="Default" w4011 {
          tunnel: [w4029 w4032] -> w4015
          tunnel: w4014 -> [w4031 _]
          tunnel: w4010 -> [w4030 w4032]
          frame Default {
            n2736 = call-poly <vilib>:"Append Waveforms.vi"("waveform B"=w4030, "waveform A"=w4031) -> ("waveform out"=w4029:waveform(dbl))  [unwired: 1 in, 8 out]
          }
          frame 1 {
          }
        }
        n2737 = feedback-in #16(w4015) -> ()
        n2738 = case shown="True" w4024 {
          tunnel: w4015 -> [_ w4028]
          frame False {
          }
          frame True {
            n2739 = call-poly <vilib>:"Mean.vi"("X"=w4028) -> ("mean"=→"Slow mean":dbl)  [unwired: 1 out]
          }
        }
      }
    }
    n2740 = Index Array(array=w3562, index=0) -> (element=w3572:waveform(dbl))
    n2741 = Index Array(array=w3562, index=1) -> (element=w3570:waveform(dbl))
    n2742 = case "For computing FFTs for display" shown="True" "Compute FFT" {
      tunnel: w3589 -> [_ w4723]
      frame False {
      }
      frame True {
        n2743 = Build Array("FFT 1 Choice 1", "FFT 1 Choice 2", "FFT 2 Choice 1", "FFT 2 Choice 2") -> (w4716:u16[])
        n2744 = Array Size(array=w4723) -> (size(s)=w4722:i32)
        n2745 = feedback-in #17(w4716) -> ()
        n2746 = feedback #17(u16[] [100, 100, 100, 100]) -> (w4717:u16[])
        n2747 = feedback-in #18("# Spectra to Ave.") -> ()
        n2748 = feedback #18("# Spectra to Ave.") -> (w4714:dbl)
        n2749 = Not Equal?(x="# Spectra to Ave.", y=w4714) -> (x != y?=w4713:bool)
        n2750 = Not Equal?(x=w4716, y=w4717) -> (x != y?=w4715:bool)
        n2751 = feedback #19(1.0) -> (w4700:dbl)
        n2752 = Compound Arithmetic op=OR("Reset FFT", w4715, w4713) -> (w4698:bool)
        n2753 = Select(t=1.0, s=w4698, f=w4700) -> (s? t:f=w4702:dbl)
        n2754 = Greater?(x=w4702, y="# Spectra to Ave.") -> (0:w4721:bool)
        n2755 = Increment(x=w4702) -> (x+1=w4701:dbl)
        n2756 = feedback-in #19(w4701) -> ()
        n2757 = local read "DMA Update Period (s)"() -> (w4696:dbl)
        n2758 = Multiply(x="# Spectra to Ave.", y=w4696) -> (x*y=→"Ave. Time (s)":dbl)
        n2759 = Build Array(cluster{"f0":dbl, "df":dbl, "magnitude":dbl[]} {"f0"=0.0, "df"=0.0, "magnitude"=[]} ("PSD")) -> (w4705:cluster{"f0":dbl, "df":dbl, "magnitude":dbl[]}[])
        n2760 = Build Array(w4705, w4705, w4705, w4705) -> (w4707:T46)
        n2761 = feedback #20(w4707) -> (w4712:T46)
        n2762 = for {
          N: 4 -> [_]
          tunnel: w4716 -> [w4745] mode=indexing
          tunnel: w4723 -> [w4746]
          tunnel: w4722 -> [w4748]
          tunnel: w4698 -> [w4741]
          tunnel: w4721 -> [w4740]
          tunnel: "# Spectra to Ave." -> [w4739]
          tunnel: [w4738] -> w4711 mode=indexing
          tunnel: w4712 -> [w4743] mode=indexing
          tunnel: [w4742] -> w4699 mode=indexing
          tunnel: w4702 -> [w4737]
          n2763 = Less?(x=w4745, y=w4748) -> (x < y?=w4747:bool)
          n2764 = Index Array(array=w4746, index=w4745) -> (element=w4744:waveform(dbl))
          n2765 = case shown="True" w4747 {
            tunnel: w4744 -> [_ w4765]
            tunnel: w4743 -> [w4750 w4763]
            tunnel: [w4750 w4751] -> w4742
            tunnel: w4741 -> [_ w4762]
            tunnel: w4740 -> [_ w4755]
            tunnel: w4739 -> [_ w4754]
            tunnel: [cluster{"f0":dbl, "df":dbl, "magnitude":dbl[]} {"f0"=0.0, "df"=0.0, "magnitude"=[]} ("PSD") w4756] -> w4738
            tunnel: w4737 -> [_ w4753]
            frame False {
            }
            frame True {
              n2766 = call <vilib>:"Std Deviation and Variance.vi"("X"=w4765) -> ("mean"=w4766:dbl)  [unwired: 1 in, 2 out]
              n2767 = Subtract(x=w4765, y=w4766) -> (x-y=w4764:waveform(dbl))
              n2768 = xnode "Spectral Measurements"("Signals"=w4764) -> ("PSD"=w4758:cluster{"f0":dbl, "df":dbl, "magnitude":dbl[]})  [unwired: 1 in, 1 out]
              n2769 = case shown="False" w4762 {
                tunnel: w4763 -> [w4775 _]
                tunnel: [w4771 w4780] -> w4751
                tunnel: w4758 -> [w4774 w4781]
                tunnel: w4755 -> [w4773 _]
                frame False {
                  n2770 = Build Array (concatenate)(w4775, w4774) -> (w4772:cluster{"f0":dbl, "df":dbl, "magnitude":dbl[]}[])
                  n2771 = case shown="True" w4773 {
                    tunnel: w4772 -> [w4776 w4779]
                    tunnel: [w4776 w4777] -> w4771
                    frame False {
                    }
                    frame True {
                      n2772 = Delete From Array(array=w4779, index=0) -> (array with subset deleted=w4777:cluster{"f0":dbl, "df":dbl, "magnitude":dbl[]}[])  [unwired: 1 in, 1 out]
                    }
                  }
                }
                frame True {
                  n2773 = Build Array(w4781) -> (w4780:cluster{"f0":dbl, "df":dbl, "magnitude":dbl[]}[])
                }
              }
              n2774 = for {
                tunnel: w4751 -> [w4770] mode=indexing
                tunnel: [w4769] -> w4761 mode=indexing
                workers-P: _ -> [_]
                n2775 = Unbundle By Name(w4770) -> ("magnitude"=w4769:dbl[])
              }
              n2776 = Transpose 2D Array(2D array=w4761) -> (transposed array=w4760:dbl[][])
              n2777 = for {
                tunnel: w4760 -> [w4768] mode=indexing
                tunnel: [w4767] -> w4759 mode=indexing
                workers-P: _ -> [_]
                n2778 = Add Array Elements(numeric array=w4768) -> (sum=w4767:dbl)
              }
              n2779 = Select(t=w4754, s=w4755, f=w4753) -> (s? t:f=w4752:dbl)
              n2780 = Divide(x=w4759, y=w4752) -> (x/y=w4757:dbl[])
              n2781 = Bundle By Name(cluster=w4758, "magnitude"=w4757) -> (w4756:cluster{"f0":dbl, "df":dbl, "magnitude":dbl[]})
            }
          }
        }
        n2782 = case shown="True" w4698 {
          tunnel: w4699 -> [w4730 w4736]
          tunnel: [w4730 w4731] -> w4697
          frame False {
          }
          frame True {
            n2783 = Array Subset(array=w4736, index (row)=0 ("index"), length (row)=4 ("length"), index (col)=0 ("index"), length (col)=1 ("length")) -> (w4731:T46)
          }
        }
        n2784 = feedback-in #20(w4697) -> ()
        n2785 = Split 1D Array(array=w4711, index=2) -> (first subarray=→"FFT 1":cluster{"f0":dbl, "df":dbl, "magnitude":dbl[]}[], second subarray=→"FFT 2":cluster{"f0":dbl, "df":dbl, "magnitude":dbl[]}[])
      }
    }
    n2786 = case "For plotting results of scanning MCL" shown="True" w3703 {
      tunnel: w3702 -> [_ w4149]
      tunnel: w3620 -> [_ w4245]
      tunnel: w3711 -> [_ _]
      tunnel: w3589 -> [_ w4219]
      tunnel: w3564 -> [_ w4150]
      tunnel: w3563 -> [_ w4123]
      frame False {
      }
      frame True {
        w4130 = u32 0 items=["Horizontal", "Vertical", "Central", "1st Diagonal", "2nd Diagonal"] ("Type of Symmetry")
        w4158 = u32 0 items=["Horizontal", "Vertical", "Central", "1st Diagonal", "2nd Diagonal"] ("Type of Symmetry")
        w4161 = u32 0 items=["Horizontal", "Vertical", "Central", "1st Diagonal", "2nd Diagonal"] ("Type of Symmetry")
        w4190 = u32 0 items=["Horizontal", "Vertical", "Central", "1st Diagonal", "2nd Diagonal"] ("Type of Symmetry")
        n2787 = Index Array(array=w4219, index=10) -> (element=w4225:waveform(dbl))
        n2788 = Index Array(array=w4219, index=11) -> (element=w4222:waveform(dbl))
        n2789 = local read "Cycles/step (MCL)"() -> (w4175:u64)
        n2790 = Index Array(array=w4219, index="Channel") -> (element=w4221:waveform(dbl))
        n2791 = Unbundle(w4123) -> ("New Image"=w4122:T2, "New Image"=w4121:T2, "New Image"=w4120:T2, "New Image"=w4119:T2)
        n2792 = Unbundle By Name(w4225) -> ("Y"=w4177:dbl[])
        n2793 = Unbundle By Name(w4222) -> ("Y"=w4179:dbl[])
        n2794 = Unbundle By Name(w4221) -> ("Y"=w4184:dbl[])
        n2795 = call "downsample 1D array - double.vi"("Ave N"=w4175, "Array In"=w4177) -> ("Array Out"=w4176:dbl[])  [unwired: 1 out]
        n2796 = call "downsample 1D array - double.vi"("Ave N"=w4175, "Array In"=w4179) -> ("Array Out"=w4178:dbl[])  [unwired: 1 out]
        n2797 = call "downsample 1D array - double.vi"("Ave N"=w4175, "Array In"=w4184) -> ("Array Out"=w4183:dbl[])  [unwired: 1 out]
        n2798 = feedback #21(w4245) -> (w4246:dbl[])
        n2799 = Build Array (concatenate)(w4246, w4245) -> (w4227:dbl[])
        n2800 = feedback #22(w4150) -> (w4152:dbl[])
        n2801 = Build Array (concatenate)(w4152, w4150) -> (w4151:dbl[])
        n2802 = local read "Scan steps (MCL)"() -> (w4132:u64)
        n2803 = Select(t=w4245, s=w4149, f=w4227) -> (s? t:f=w4231:dbl[])
        n2804 = feedback-in #21(w4231) -> ()
        n2805 = Select(t=w4150, s=w4149, f=w4151) -> (s? t:f=w4133:dbl[])
        n2806 = feedback-in #22(w4133) -> ()
        n2807 = local read "Scan lines (y)"() -> (w4118:u64)
        n2808 = local read "N APD Samp/step"() -> (w4134:dbl)
        n2809 = feedback #23(w4176) -> (w4233:dbl[])
        n2810 = Build Array (concatenate)(w4233, w4176) -> (w4224:dbl[])
        n2811 = feedback #24(w4183) -> (w4243:dbl[])
        n2812 = Build Array (concatenate)(w4243, w4183) -> (w4242:dbl[])
        n2813 = feedback #25(w4178) -> (w4235:dbl[])
        n2814 = Build Array (concatenate)(w4235, w4178) -> (w4236:dbl[])
        n2815 = Select(t=w4176, s=w4149, f=w4224) -> (s? t:f=w4180:dbl[])
        n2816 = feedback-in #23(w4180) -> ()
        n2817 = Select(t=w4183, s=w4149, f=w4242) -> (s? t:f=w4182:dbl[])
        n2818 = feedback-in #24(w4182) -> ()
        n2819 = Select(t=w4178, s=w4149, f=w4236) -> (s? t:f=w4181:dbl[])
        n2820 = feedback-in #25(w4181) -> ()
        n2821 = Multiply(x=w4132, y=u64 2) -> (x*y=w4117:u64)
        n2822 = call "integrate 1D array interval - double.vi"("Ave N"=w4134, "Array In"=w4133) -> ("Array Out"=w4145:dbl[])  [unwired: 1 out]
        n2823 = call "integrate 1D array interval - double.vi"("Ave N"=w4134, "Array In"=w4231) -> ("Array Out"=w4230:dbl[])  [unwired: 1 out]
        n2824 = Array Size(array=w4145) -> (size(s)=w4146:i32)
        n2825 = Array Size(array=w4230) -> (size(s)=w4232:i32)
        n2826 = Multiply(x=w4118, y=w4117) -> (x*y=w4148:u64)
        n2827 = Multiply(x=w4118, y=w4117) -> (x*y=w4240:u64)
        n2828 = call-poly <vilib>:"Mean.vi"("X"=w4180) -> ("mean"=w4164:dbl)  [unwired: 1 out]
        n2829 = Subtract(x=w4148, y=w4146) -> (x-y=w4139:u64)
        n2830 = call-poly <vilib>:"Mean.vi"("X"=w4182) -> ("mean"=w4169:dbl)  [unwired: 1 out]
        n2831 = call-poly <vilib>:"Mean.vi"("X"=w4181) -> ("mean"=w4167:dbl)  [unwired: 1 out]
        n2832 = call-poly <vilib>:"Mean.vi"("X"=w4145) -> ("mean"=w4136:dbl)  [unwired: 1 out]
        n2833 = Subtract(x=w4240, y=w4232) -> (x-y=w4174:u64)
        n2834 = call-poly <vilib>:"Mean.vi"("X"=w4230) -> ("mean"=w4171:dbl)  [unwired: 1 out]
        n2835 = Initialize Array(1.0 ("element"), w4139) -> (w4135:dbl[])
        n2836 = Initialize Array(1.0 ("element"), w4174) -> (w4165:dbl[])
        n2837 = Multiply(x=w4135, y=w4136) -> (x*y=w4137:dbl[])
        n2838 = Multiply(x=w4165, y=w4167) -> (x*y=w4168:dbl[])
        n2839 = Multiply(x=w4165, y=w4169) -> (x*y=w4170:dbl[])
        n2840 = Multiply(x=w4165, y=w4164) -> (x*y=w4166:dbl[])
        n2841 = Multiply(x=w4165, y=w4171) -> (x*y=w4172:dbl[])
        n2842 = Build Array (concatenate)(w4180, w4166) -> (w4234:dbl[])
        n2843 = Build Array (concatenate)(w4182, w4170) -> (w4238:dbl[])
        n2844 = Build Array (concatenate)(w4181, w4168) -> (w4237:dbl[])
        n2845 = Build Array (concatenate)(w4145, w4137) -> (w4147:dbl[])
        n2846 = Build Array (concatenate)(w4230, w4172) -> (w4239:dbl[])
        n2847 = Reshape Array(w4234, w4118, w4117) -> (w4200:dbl[][])
        n2848 = Reshape Array(w4147, w4118, w4117) -> (w4143:dbl[][])
        n2849 = Reshape Array(w4238, w4118, w4117) -> (w4192:dbl[][])
        n2850 = Reshape Array(w4237, w4118, w4117) -> (w4207:dbl[][])
        n2851 = Reshape Array(w4239, w4118, w4117) -> (w4217:dbl[][])
        n2852 = Array Subset(array=w4207, index (col)=0 ("index"), length (col)=w4132) -> (w4212:dbl[][])  [unwired: 2 in]
        n2853 = Array Subset(array=w4207, index (col)=w4132) -> (w4210:dbl[][])  [unwired: 3 in]
        n2854 = Array Subset(array=w4192, index (col)=0 ("index"), length (col)=w4132) -> (w4198:dbl[][])  [unwired: 2 in]
        n2855 = Array Subset(array=w4192, index (col)=w4132) -> (w4196:dbl[][])  [unwired: 3 in]
        n2856 = Array Subset(array=w4143, index (col)=0 ("index"), length (col)=w4132) -> (w4142:dbl[][])  [unwired: 2 in]
        n2857 = Array Subset(array=w4143, index (col)=w4132) -> (w4140:dbl[][])  [unwired: 3 in]
        n2858 = Array Subset(array=w4217, index (col)=0 ("index"), length (col)=w4132) -> (w4216:dbl[][])  [unwired: 2 in]
        n2859 = Array Subset(array=w4217, index (col)=w4132) -> (w4214:dbl[][])  [unwired: 3 in]
        n2860 = Array Subset(array=w4200, index (col)=0 ("index"), length (col)=w4132) -> (w4205:dbl[][])  [unwired: 2 in]
        n2861 = Array Subset(array=w4200, index (col)=w4132) -> (w4203:dbl[][])  [unwired: 3 in]
        n2862 = for {
          tunnel: w4212 -> [w4254] mode=indexing
          tunnel: [w4253] -> w4211 mode=indexing
          workers-P: _ -> [_]
          n2863 = Reverse 1D Array(array=w4254) -> (reversed array=w4253:dbl[])
        }
        n2864 = for {
          tunnel: w4198 -> [w4250] mode=indexing
          tunnel: [w4249] -> w4197 mode=indexing
          workers-P: _ -> [_]
          n2865 = Reverse 1D Array(array=w4250) -> (reversed array=w4249:dbl[])
        }
        n2866 = for {
          tunnel: w4142 -> [w4248] mode=indexing
          tunnel: [w4247] -> w4141 mode=indexing
          workers-P: _ -> [_]
          n2867 = Reverse 1D Array(array=w4248) -> (reversed array=w4247:dbl[])
        }
        n2868 = for {
          tunnel: w4216 -> [w4256] mode=indexing
          tunnel: [w4255] -> w4215 mode=indexing
          workers-P: _ -> [_]
          n2869 = Reverse 1D Array(array=w4256) -> (reversed array=w4255:dbl[])
        }
        n2870 = for {
          tunnel: w4205 -> [w4252] mode=indexing
          tunnel: [w4251] -> w4204 mode=indexing
          workers-P: _ -> [_]
          n2871 = Reverse 1D Array(array=w4252) -> (reversed array=w4251:dbl[])
        }
        n2872 = Index Array(array=w4217, index (row)=0) -> (element=→"Waveform Graph":dbl[])  [unwired: 1 in]
        n2873 = Add(x=w4211, y=w4210) -> (x+y=w4209:dbl[][])
        n2874 = Add(x=w4197, y=w4196) -> (x+y=w4195:dbl[][])
        n2875 = Add(x=w4141, y=w4140) -> (x+y=w4125:dbl[][])
        n2876 = Add(x=w4215, y=w4214) -> (x+y=w4189:dbl[][])
